vi "IsCaseAvailable__slk_mt.vi"(8 "error in (no error)":errorcluster, 11 "case refnum in":refnum<vi>) -> (0 "error out":errorcluster, 3 "available?":bool)   [LabVIEW 2010, in "Lazyboots Menu Tool.lvlib"]
doc: "Check if the case is available for operations."
uses:
  Library/Lazyboots Menu Tool.lvlib
panel:
  # "IsCaseAvailable__slk_mt.vi\nCheck if the case is available for operations.\n\nNOTICE -- YOU MUST LEAVE THIS NOTICE IN PLACE.\n\nCopyright (c) 2011, LIANG LIU Shawn.Liu.cn@gmail.com\nAll rights reserved.\n\nRedistribution and use in source and binary forms, with or without modification, are permitted provided that the following conditions are met:\n-Redistributions of source code must retain the above copyright notice, this list of conditions and the following disclaimer.\n-Redistributions in binary form must reproduce the above copyright notice, this list of conditions and the following disclaimer in the documentation and/or other materials provided with the distribution.\n-Neither the name of the eLp nor the names of its contributors may be used to endorse or promote products derived from this software without specific prior written permission.\n\nTHIS SOFTWARE IS PROVIDED BY THE COPYRIGHT HOLDERS AND CONTRIBUTORS \"AS IS\" AND ANY EXPRESS OR IMPLIED WARRANTIES, INCLUDING, BUT NOT LIMITED TO, THE IMPLIED WARRANTIES OF MERCHANTABILITY AND FITNESS FOR A PARTICULAR PURPOSE ARE DISCLAIMED. IN NO EVENT SHALL THE COPYRIGHT HOLDER OR CONTRIBUTORS BE LIABLE FOR ANY DIRECT, INDIRECT, INCIDENTAL, SPECIAL, EXEMPLARY, OR CONSEQUENTIAL DAMAGES (INCLUDING, BUT NOT LIMITED TO, PROCUREMENT OF SUBSTITUTE GOODS OR SERVICES; LOSS OF USE, DATA, OR PROFITS; OR BUSINESS INTERRUPTION) HOWEVER CAUSED AND ON ANY THEORY OF LIABILITY, WHETHER IN CONTRACT, STRICT LIABILITY, OR TORT (INCLUDING NEGLIGENCE OR OTHERWISE) ARISING IN ANY WAY OUT OF THE USE OF THIS SOFTWARE, EVEN IF ADVISED OF THE POSSIBILITY OF SUCH DAMAGE."
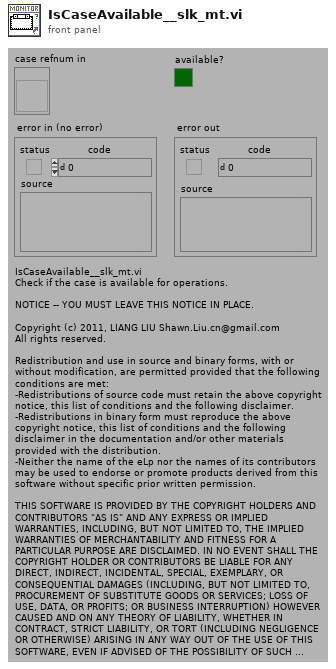
[diagram p1: front panel]
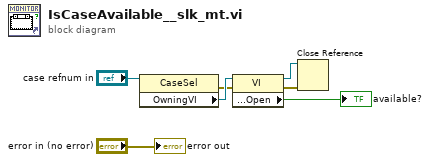
[diagram p0: block diagram]
diagram:
  n1 = property class="CaseSel"(reference="case refnum in") -> (error out=w3:errorcluster, "OwningVI"=w5:refnum<vi>)  [unwired: 1 in, 1 out]
  n2 = property class="VI"(reference=w5, error in=w3) -> (reference out=w1:refnum<vi>, error out=w2:errorcluster, "Front Panel.Open"=→"available?":bool)
  n3 = Close Reference(reference=w1, error in (no error)=w2) -> ()  [unwired: 1 out]
  "error out" <- "error in (no error)"
